vi "Update.vi"(8 "error in (no error)":errorcluster, 10 "Message in":refnum<class "UpdateMessage.lvclass">, 11 "Galvo in":refnum<class "InVivo_ImagingModeSPIM.lvclass">) -> (0 "error out":errorcluster, 3 "Galvo out":refnum<class "InVivo_ImagingModeSPIM.lvclass">)   [LabVIEW 2012, in "InVivo_ImagingModeSPIM.lvclass"]
doc: "The update method processes the command 'update'. \n\nThe command 'update' is used for receiving new values to be set to the private data of the class. This could be seen as a public set method for setting new parameters to the private class data."
uses:
  InVivo_ImagingModeSPIM.lvclass
  <vilib>/Distrio/Murmex/UpdateMessage/UpdateMessage.lvclass
  InVivo_ImagingModeSPIM.lvclass/InVivo_ImagingModeSPIM.ctl
  Controls/waveform_enum.ctl
  Control 4.ctl
  <vilib>/Distrio/Murmex/Murmex/Murmex.lvclass
panel:
  # "This method is called when the UPDATE\ntrigger is sent. \n\nOverride this method when your component needs to\nrespond to this trigger. \n\nCall parent for proper implementation"
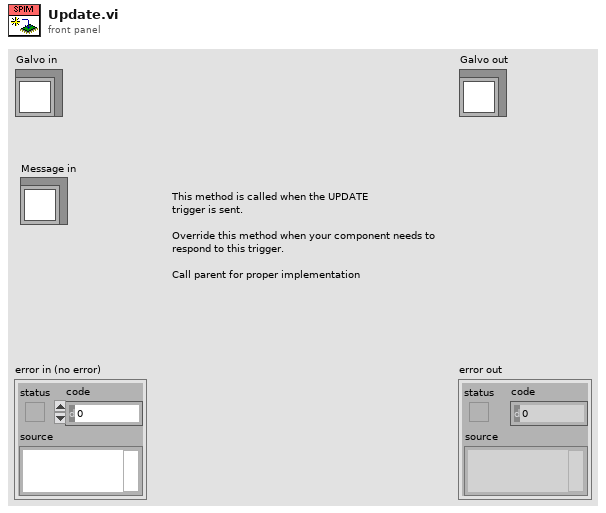
[diagram p1: front panel]
types:
  T1 = typedef "InVivo_ImagingModeSPIM.lvclass/waveform_enum.ctl" = enum16{"triangular", "sawtooth", "sinusodial"}
  T2 = typedef "InVivo_ImagingModeSPIM.lvclass/Control 4.ctl" = enum16{"Triangular", "Sawtooth", "Sinusoidal"}
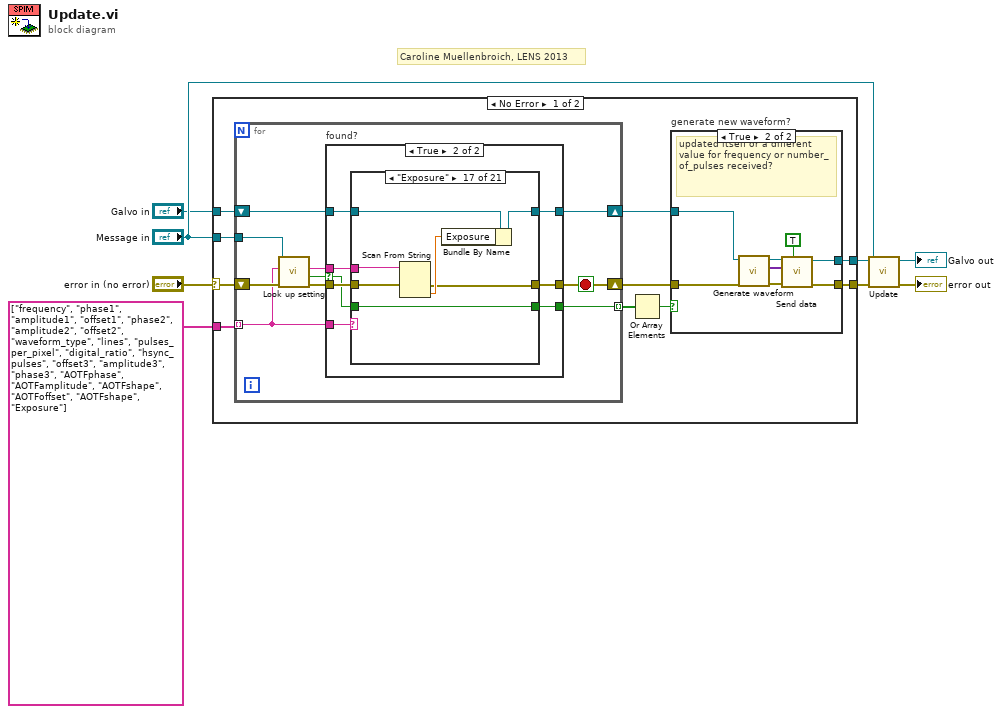
[diagram p0: block diagram]
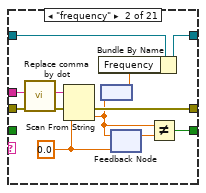
[diagram p5: hidden frame]
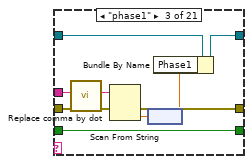
[diagram p6: hidden frame]
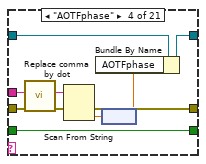
[diagram p7: hidden frame]
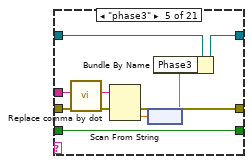
[diagram p8: hidden frame]
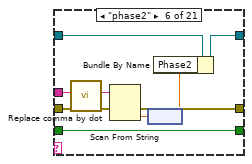
[diagram p9: hidden frame]
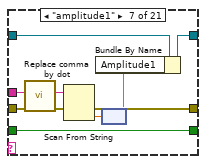
[diagram p10: hidden frame]
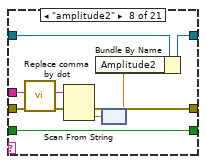
[diagram p11: hidden frame]
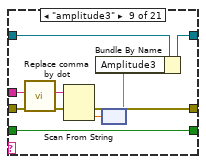
[diagram p12: hidden frame]
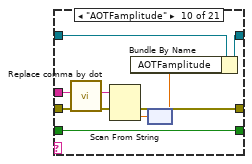
[diagram p13: hidden frame]
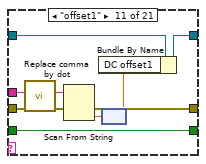
[diagram p14: hidden frame]
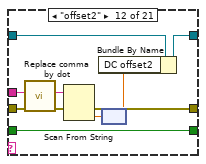
[diagram p15: hidden frame]
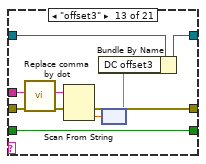
[diagram p16: hidden frame]
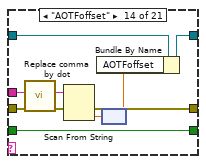
[diagram p17: hidden frame]
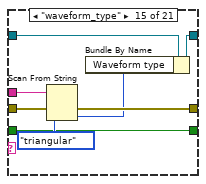
[diagram p18: hidden frame]
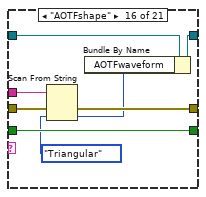
[diagram p19: hidden frame]
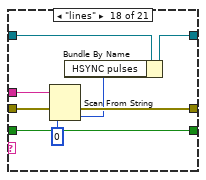
[diagram p20: hidden frame]
diagram:
  # "Caroline Muellenbroich, LENS 2013"
  n1 = case shown="No Error" "error in (no error)" {
    selector: "error in (no error)" -> [w18 w228]
    tunnel: [w13 w229] -> w5
    tunnel: "Galvo in" -> [w11 w229]
    tunnel: [w12 w228] -> w4
    tunnel: "Message in" -> [w17 _]
    tunnel: string[] ["frequency", "phase1", "amplitude1", "offset1", "phase2", "amplitude2", "offset2", "waveform_type", "lines", "pulses_per_pixel", "digital_ratio", "hsync_pulses", "offset3", "amplitude3", "phase3", "AOTFphase", "AOTFamplitude", "AOTFshape", "AOTFoffset", "AOTFshape", "Exposure"] ("key chains") -> [w14 _]
    frame No Error {
      n2 = for {
        tunnel: w17 -> [w37]
        tunnel: w14 -> [w30] mode=indexing
        shift-right: [w31] -> w16
        shift-left: w18 -> [w38]
        shift-right: [w33] -> w15
        shift-left: w11 -> [w34]
        tunnel: [w29] -> w10 mode=indexing
        stop <- w31 stop-if-true
        n3 = call <vilib>:"Look up setting.vi"("error in (no error)"=w38, "tag name"=w30, "UpdateMessage in"=w37) -> ("error out"=w35:errorcluster, "found?"=w36:bool, "value"=w32:string)  [unwired: 5 in, 1 out]
        n4 = case "found?" shown="True" w36 {
          selector: w36 -> [w39 w42]
          tunnel: w35 -> [w41 w47]
          tunnel: [w41 w48] -> w31
          tunnel: w34 -> [w40 w45]
          tunnel: [w40 w46] -> w33
          tunnel: w32 -> [_ w44]
          tunnel: w30 -> [_ w49]
          tunnel: [w39 w43] -> w29
          frame False {
          }
          frame True {
            n5 = case shown="\"Exposure\"" w49 {
              tunnel: w44 -> [_ w62 w71 w80 w89 w98 w107 w116 w125 w134 w143 w152 w161 w170 w176 w184 w193 w198 w206 w215 w226]
              tunnel: [w52 w60 w69 w78 w87 w96 w105 w114 w123 w132 w141 w150 w159 w168 w175 w183 w188 w199 w207 w216 w224] -> w48
              tunnel: w47 -> [w52 w63 w72 w81 w90 w99 w108 w117 w126 w135 w144 w153 w162 w171 w177 w185 w189 w200 w208 w217 w227]
              tunnel: [w51 w59 w66 w75 w84 w93 w102 w111 w120 w129 w138 w147 w156 w165 w178 w186 w191 w201 w209 w218 w223] -> w46
              tunnel: w45 -> [w51 w61 w70 w79 w88 w97 w106 w115 w124 w133 w142 w151 w160 w169 w179 w187 w192 w202 w210 w219 w225]
              tunnel: [w50 w53 w64 w73 w82 w91 w100 w109 w118 w127 w136 w145 w154 w163 w172 w181 w194 w195 w203 w211 w220] -> w43
              tunnel: w42 -> [w50 _ w64 w73 w82 w91 w100 w109 w118 w127 w136 w145 w154 w163 w172 w181 w194 w195 w203 _ w220]
              frame Default {
              }
              frame "frequency" {
                w55 = 0.0 ("default value 1")
                n6 = call <vilib>:"Replace comma by dot.vi"("input string"=w62) -> ("result string"=w58:string)  [unwired: 10 in]
                n7 = Scan From String(input string=w58, error in=w63, default 1=w55) -> (error out=w60:errorcluster, output 1=w54:dbl)  [unwired: 2 in, 2 out]
                n8 = node(w54) -> (w57:dbl[unit])
                n9 = Bundle By Name(cluster=w61, "Frequency"=w57) -> (w59:refnum<class "InVivo_ImagingModeSPIM.lvclass">)
                n10 = feedback #1(w55) -> (w56:dbl)
                n11 = feedback-in #1(w54) -> ()
                n12 = Not Equal?(x=w54, y=w56) -> (x != y?=w53:bool)
              }
              frame "phase1" {
                n13 = call <vilib>:"Replace comma by dot.vi"("input string"=w71) -> ("result string"=w65:string)  [unwired: 10 in]
                n14 = Scan From String(input string=w65, error in=w72) -> (error out=w69:errorcluster, output 1=w68:dbl)  [unwired: 3 in, 2 out]
                n15 = node(w68) -> (w67:dbl[unit])
                n16 = Bundle By Name(cluster=w70, "Phase1"=w67) -> (w66:refnum<class "InVivo_ImagingModeSPIM.lvclass">)
              }
              frame "AOTFphase" {
                n17 = call <vilib>:"Replace comma by dot.vi"("input string"=w80) -> ("result string"=w74:string)  [unwired: 10 in]
                n18 = Scan From String(input string=w74, error in=w81) -> (error out=w78:errorcluster, output 1=w77:dbl)  [unwired: 3 in, 2 out]
                n19 = node(w77) -> (w76:dbl[unit])
                n20 = Bundle By Name(cluster=w79, "AOTFphase"=w76) -> (w75:refnum<class "InVivo_ImagingModeSPIM.lvclass">)
              }
              frame "phase3" {
                n21 = call <vilib>:"Replace comma by dot.vi"("input string"=w89) -> ("result string"=w83:string)  [unwired: 10 in]
                n22 = Scan From String(input string=w83, error in=w90) -> (error out=w87:errorcluster, output 1=w86:dbl)  [unwired: 3 in, 2 out]
                n23 = node(w86) -> (w85:dbl[unit])
                n24 = Bundle By Name(cluster=w88, "Phase3"=w85) -> (w84:refnum<class "InVivo_ImagingModeSPIM.lvclass">)
              }
              frame "phase2" {
                n25 = call <vilib>:"Replace comma by dot.vi"("input string"=w98) -> ("result string"=w92:string)  [unwired: 10 in]
                n26 = Scan From String(input string=w92, error in=w99) -> (error out=w96:errorcluster, output 1=w95:dbl)  [unwired: 3 in, 2 out]
                n27 = node(w95) -> (w94:dbl[unit])
                n28 = Bundle By Name(cluster=w97, "Phase2"=w94) -> (w93:refnum<class "InVivo_ImagingModeSPIM.lvclass">)
              }
              frame "amplitude1" {
                n29 = call <vilib>:"Replace comma by dot.vi"("input string"=w107) -> ("result string"=w101:string)  [unwired: 10 in]
                n30 = Scan From String(input string=w101, error in=w108) -> (error out=w105:errorcluster, output 1=w104:dbl)  [unwired: 3 in, 2 out]
                n31 = node(w104) -> (w103:dbl[unit])
                n32 = Bundle By Name(cluster=w106, "Amplitude1"=w103) -> (w102:refnum<class "InVivo_ImagingModeSPIM.lvclass">)
              }
              frame "amplitude2" {
                n33 = call <vilib>:"Replace comma by dot.vi"("input string"=w116) -> ("result string"=w110:string)  [unwired: 10 in]
                n34 = Scan From String(input string=w110, error in=w117) -> (error out=w114:errorcluster, output 1=w113:dbl)  [unwired: 3 in, 2 out]
                n35 = node(w113) -> (w112:dbl[unit])
                n36 = Bundle By Name(cluster=w115, "Amplitude2"=w112) -> (w111:refnum<class "InVivo_ImagingModeSPIM.lvclass">)
              }
              frame "amplitude3" {
                n37 = call <vilib>:"Replace comma by dot.vi"("input string"=w125) -> ("result string"=w119:string)  [unwired: 10 in]
                n38 = Scan From String(input string=w119, error in=w126) -> (error out=w123:errorcluster, output 1=w122:dbl)  [unwired: 3 in, 2 out]
                n39 = node(w122) -> (w121:dbl[unit])
                n40 = Bundle By Name(cluster=w124, "Amplitude3"=w121) -> (w120:refnum<class "InVivo_ImagingModeSPIM.lvclass">)
              }
              frame "AOTFamplitude" {
                n41 = call <vilib>:"Replace comma by dot.vi"("input string"=w134) -> ("result string"=w128:string)  [unwired: 10 in]
                n42 = Scan From String(input string=w128, error in=w135) -> (error out=w132:errorcluster, output 1=w131:dbl)  [unwired: 3 in, 2 out]
                n43 = node(w131) -> (w130:dbl[unit])
                n44 = Bundle By Name(cluster=w133, "AOTFamplitude"=w130) -> (w129:refnum<class "InVivo_ImagingModeSPIM.lvclass">)
              }
              frame "offset1" {
                n45 = call <vilib>:"Replace comma by dot.vi"("input string"=w143) -> ("result string"=w137:string)  [unwired: 10 in]
                n46 = Scan From String(input string=w137, error in=w144) -> (error out=w141:errorcluster, output 1=w140:dbl)  [unwired: 3 in, 2 out]
                n47 = node(w140) -> (w139:dbl[unit])
                n48 = Bundle By Name(cluster=w142, "DC offset1"=w139) -> (w138:refnum<class "InVivo_ImagingModeSPIM.lvclass">)
              }
              frame "offset2" {
                n49 = call <vilib>:"Replace comma by dot.vi"("input string"=w152) -> ("result string"=w146:string)  [unwired: 10 in]
                n50 = Scan From String(input string=w146, error in=w153) -> (error out=w150:errorcluster, output 1=w149:dbl)  [unwired: 3 in, 2 out]
                n51 = node(w149) -> (w148:dbl[unit])
                n52 = Bundle By Name(cluster=w151, "DC offset2"=w148) -> (w147:refnum<class "InVivo_ImagingModeSPIM.lvclass">)
              }
              frame "offset3" {
                n53 = call <vilib>:"Replace comma by dot.vi"("input string"=w161) -> ("result string"=w155:string)  [unwired: 10 in]
                n54 = Scan From String(input string=w155, error in=w162) -> (error out=w159:errorcluster, output 1=w158:dbl)  [unwired: 3 in, 2 out]
                n55 = node(w158) -> (w157:dbl[unit])
                n56 = Bundle By Name(cluster=w160, "DC offset3"=w157) -> (w156:refnum<class "InVivo_ImagingModeSPIM.lvclass">)
              }
              frame "AOTFoffset" {
                n57 = call <vilib>:"Replace comma by dot.vi"("input string"=w170) -> ("result string"=w164:string)  [unwired: 10 in]
                n58 = Scan From String(input string=w164, error in=w171) -> (error out=w168:errorcluster, output 1=w167:dbl)  [unwired: 3 in, 2 out]
                n59 = node(w167) -> (w166:dbl[unit])
                n60 = Bundle By Name(cluster=w169, "AOTFoffset"=w166) -> (w165:refnum<class "InVivo_ImagingModeSPIM.lvclass">)
              }
              frame "waveform_type" {
                n61 = Scan From String(input string=w176, error in=w177, default 1=waveform_enum."triangular" ("Waveform type")) -> (error out=w175:errorcluster, output 1=w173:T1)  [unwired: 2 in, 2 out]
                n62 = Bundle By Name(cluster=w179, "Waveform type"=w173) -> (w178:refnum<class "InVivo_ImagingModeSPIM.lvclass">)
              }
              frame "AOTFshape" {
                n63 = Scan From String(input string=w184, error in=w185, default 1=Control_4."Triangular" ("AOTFwaveform")) -> (error out=w183:errorcluster, output 1=w182:T2)  [unwired: 2 in, 2 out]
                n64 = Bundle By Name(cluster=w187, "AOTFwaveform"=w182) -> (w186:refnum<class "InVivo_ImagingModeSPIM.lvclass">)
              }
              frame "Exposure" {
                n65 = Scan From String(input string=w193, error in=w189) -> (error out=w188:errorcluster, output 1=w190:dbl)  [unwired: 3 in, 2 out]
                n66 = Bundle By Name(cluster=w192, "Exposure"=w190) -> (w191:refnum<class "InVivo_ImagingModeSPIM.lvclass">)
              }
              frame "lines" {
                n67 = Scan From String(input string=w198, error in=w200, default 1=0) -> (error out=w199:errorcluster, output 1=w196:i32)  [unwired: 2 in, 2 out]
                n68 = Bundle By Name(cluster=w202, "HSYNC pulses"=w196) -> (w201:refnum<class "InVivo_ImagingModeSPIM.lvclass">)
              }
              frame "pulses_per_pixel" {
                n69 = Scan From String(input string=w206, error in=w208, default 1=0) -> (error out=w207:errorcluster, output 1=w204:i32)  [unwired: 2 in, 2 out]
                n70 = Bundle By Name(cluster=w210, "pulses per pixel"=w204) -> (w209:refnum<class "InVivo_ImagingModeSPIM.lvclass">)
              }
              frame "hsync_pulses" {
                w212 = 0
                n71 = Scan From String(input string=w215, error in=w217, default 1=w212) -> (error out=w216:errorcluster, output 1=w214:i32)  [unwired: 2 in, 2 out]
                n72 = Bundle By Name(cluster=w219, "HSYNC pulses"=w214) -> (w218:refnum<class "InVivo_ImagingModeSPIM.lvclass">)
                n73 = feedback-in #2(w214) -> ()
                n74 = feedback #2(w212) -> (w213:i32)
                n75 = Not Equal?(x=w214, y=w213) -> (x != y?=w211:bool)
              }
              frame "digital_ratio" {
                n76 = call <vilib>:"Replace comma by dot.vi"("input string"=w226) -> ("result string"=w222:string)  [unwired: 10 in]
                n77 = Scan From String(input string=w222, error in=w227) -> (error out=w224:errorcluster, output 1=w221:dbl)  [unwired: 3 in, 2 out]
                n78 = Bundle By Name(cluster=w225, "digital ratio"=w221) -> (w223:refnum<class "InVivo_ImagingModeSPIM.lvclass">)
              }
            }
          }
        }
      }
      n79 = Or Array Elements(Boolean array=w10) -> (logical OR=w9:bool)
      n80 = case "generate new waveform?" shown="True" w9 {
        tunnel: w16 -> [w19 w24]
        tunnel: w15 -> [w20 w25]
        tunnel: [w20 w28] -> w13
        tunnel: [w19 w27] -> w12
        frame False {
        }
        frame True {
          # "updated itself or a different value for frequency or number_of_pulses received?"
          n81 = call-dynamic "Generate waveform.vi"("error in (no error)"=w24, "Galvo in"=w25) -> ("error out"=w21:errorcluster, "Array"=w22:variant[], "Galvo out"=w23:refnum<class "InVivo_ImagingModeSPIM.lvclass">)  [unwired: 7 in]
          n82 = call <vilib>:"Send data.vi"("is finalised data? (T)"=TRUE, "error in (no error)"=w21, "data (channels array)"=w22, "Murmex in"=w23) -> ("error out"=w27:errorcluster, "Murmex out"=w28:refnum<class "InVivo_ImagingModeSPIM.lvclass">)  [unwired: 6 in]
        }
      }
    }
    frame Error {
    }
  }
  n83 = call-parent "Update.vi"("error in (no error)"=w4, "Message in"="Message in", "Murmex in"=w5) -> ("error out"=→"error out":errorcluster, "Murmex out"=→"Galvo out":refnum<class "InVivo_ImagingModeSPIM.lvclass">)  [unwired: 7 in]
